vi "Host - Download.vi"(8 "Error In (no error)":errorcluster, 9 "bitfile path in":path, 11 "Slave Ref in":refnum<k21>) -> (0 "error out":errorcluster, 1 "bitfile path out":path, 3 "Slave Ref out":refnum<k21>)   [LabVIEW 2016, in "Scan Engine Custom Device.lvlib"]
uses:
  Scan Engine Custom Device.lvlib
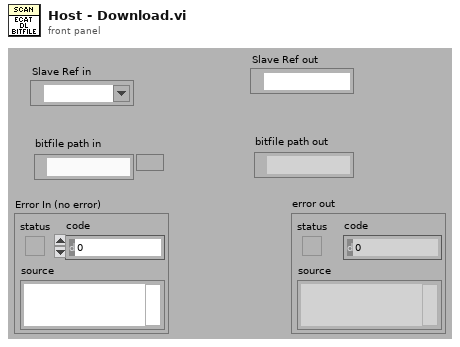
[diagram p1: front panel]
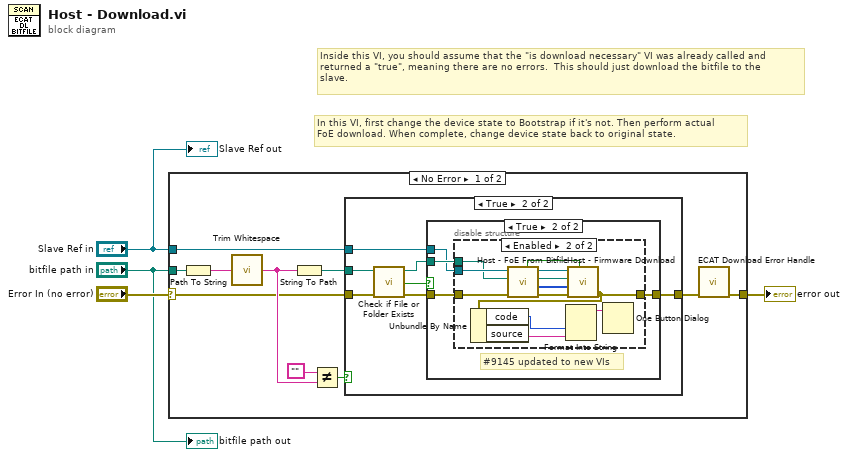
[diagram p0: block diagram]
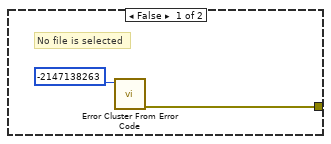
[diagram p2: hidden frame]
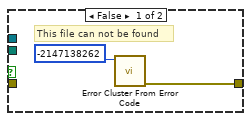
[diagram p3: hidden frame]
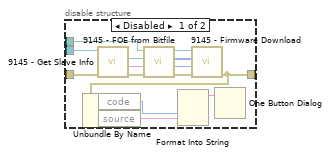
[diagram p4: hidden frame]
diagram:
  # "In this VI, first change the device state to Bootstrap if it's not. Then perform actual\nFoE download. When complete, change device state back to original state."
  # "Inside this VI, you should assume that the \"is download necessary\" VI was already called and\nreturned a \"true\", meaning there are no errors.  This should just download the bitfile to the\nslave."
  n1 = case shown="No Error" "Error In (no error)" {
    selector: "Error In (no error)" -> [w6 w56]
    tunnel: [w14 w56] -> w4
    tunnel: "bitfile path in" -> [w8 _]
    tunnel: "Slave Ref in" -> [w7 _]
    frame No Error {
      n2 = Path To String(path=w8) -> (string=w11:string)
      n3 = call <vilib>:"Trim Whitespace.vi"("string"=w11) -> ("trimmed string"=w13:string)  [unwired: 1 in]
      n4 = String To Path(string=w13) -> (path=w9:path)
      n5 = Not Equal?(x="", y=w13) -> (x != y?=w10:bool)
      n6 = case shown="True" w10 {
        tunnel: w7 -> [_ w23]
        tunnel: w9 -> [_ w22]
        tunnel: [w15 w18] -> w5
        tunnel: w6 -> [_ w17]
        frame False {
          # "No file is selected"
          n7 = call <vilib>:"Error Cluster From Error Code.vi"("error code (0)"=-2147138263) -> ("error out"=w15:errorcluster)  [unwired: 8 in]
        }
        frame True {
          n8 = call <vilib>:"Check if File or Folder Exists.vi"("error in (no error)"=w17, "path"=w22) -> ("error out"=w19:errorcluster, "file or folder exists?"=w21:bool, "dup path"=w20:path)  [unwired: 7 out]
          n9 = case shown="True" w21 {
            tunnel: w23 -> [_ w27]
            tunnel: w20 -> [_ w28]
            tunnel: w19 -> [_ w29]
            tunnel: [w24 w26] -> w18
            frame False {
              # "This file can not be found"
              n10 = call <vilib>:"Error Cluster From Error Code.vi"("error code (0)"=-2147138262) -> ("error out"=w24:errorcluster)  [unwired: 8 in]
            }
            frame True {
              # "#9145 updated to new VIs"
              n11 = disable-structure shown="Enabled" {
                disable-tunnel: w29 -> [w43 w55]
                disable-tunnel: w28 -> [w35 w48]
                disable-tunnel: w27 -> [w34 w49]
                disable-tunnel: [w33 w45] -> w26
                frame Disabled {
                  n12 = call "9145 - Get Slave Info.vi"("error in (no error)"=w43, "Slave Ref in"=w34) -> ("error out"=w42:errorcluster, "IP Address"=w37:string, "NI-ECAT Slave Ref out"=w36:refnum<k21>)  [unwired: 7 in]
                  n13 = call "9145 - FOE from Bitfile.vi"("error in (no error)"=w42, "IP Address"=w37, "NI-ECAT Slave Ref In"=w36, "Firmware filename"=w35) -> ("error out"=w41:errorcluster, "hServer Out"=w40:u64, "File Byte Array"=w39:u8[], "NI-ECAT Slave Ref Out"=w38:refnum<k21>)  [unwired: 4 in]
                  n14 = call "9145 - Firmware Download.vi"("Error In"=w41, "hServer In"=w40, "File Byte Array"=w39, "Slave Ref In"=w38) -> ("error out"=w33:errorcluster)  [unwired: 7 in]
                  n15 = Unbundle By Name(w33) -> ("code"=w32:i32, "source"=w30:string)
                  n16 = Format Into String(w32, w30) -> (resulting string=w31:string)  [unwired: 3 in, 1 out]
                  n17 = One Button Dialog(message=w31) -> ()  [unwired: 1 in, 1 out]
                }
                frame Enabled {
                  n18 = call "Host - FoE From Bitfile.vi"("error in (no error)"=w55, "Firmware filename"=w48, "Slave Ref in"=w49) -> ("error out"=w54:errorcluster, "File Byte Array"=w53:u8[], "Firmware filename out"=w52:path, "Slave Ref out"=w51:refnum<k21>, "Need Reset"=w50:bool)  [unwired: 4 in]
                  n19 = call "Host - Firmware Download.vi"("Need Reset"=w50, "error in (no error)"=w54, "File Byte Array"=w53, "Firmware filename"=w52, "Slave Ref in"=w51) -> ("error out"=w45:errorcluster)  [unwired: 6 in]
                  n20 = Unbundle By Name(w45) -> ("code"=w47:i32, "source"=w44:string)
                  n21 = Format Into String(w47, w44) -> (resulting string=w46:string)  [unwired: 3 in, 1 out]
                  n22 = One Button Dialog(message=w46) -> ()  [unwired: 1 in, 1 out]
                }
              }
            }
          }
        }
      }
      n23 = call "ECAT Download Error Handle.vi"("error in"=w5) -> ("error out"=w14:errorcluster)  [unwired: 10 in]
    }
    frame Error {
    }
  }
  "error out" <- w4
  "bitfile path out" <- "bitfile path in"
  "Slave Ref out" <- "Slave Ref in"
